vi "Read-state.vi"(8 "error in (no error)":errorcluster, 11 "Plant":enum16{"Plant 1", "Plant 2"}(ring)) -> (0 "error out":errorcluster, 2 "state":dbl[](array[numeric]) caption="data" format="%.2f")   [LabVIEW 2016]
uses:
  <vilib>/xnet/xnet.llb/XNET Read (Signal Single-point).vi
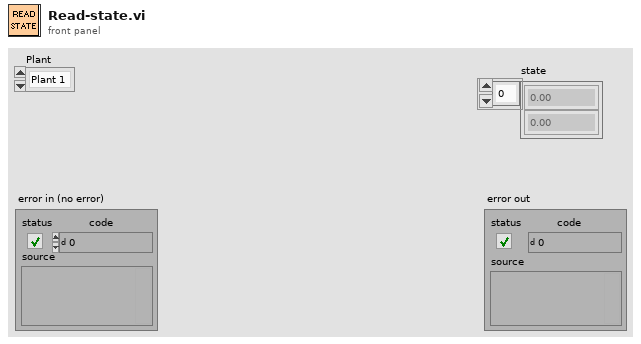
[diagram p1: front panel]
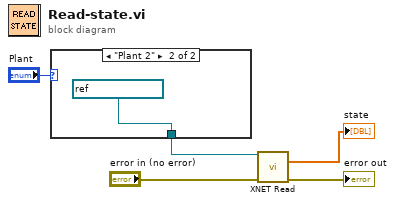
[diagram p0: block diagram]
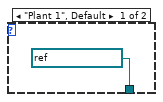
[diagram p2: hidden frame]
diagram:
  n1 = case shown="\"Plant 2\"" "Plant" {
    tunnel: [refnum<k21> "Plant1_state" ("session in") refnum<k21> "Plant2_state" ("session in")] -> w1
    frame "Plant 1", Default {
    }
    frame "Plant 2" {
    }
  }
  n2 = call-poly <vilib>:"XNET Read.vi"("session in"=w1, "error in (no error)"="error in (no error)") -> ("data"=→"state":dbl[], "error out"=→"error out":errorcluster)  [unwired: 11 in, 1 out]
